vi "Get Indicators.vi"(6 "Indicator Names":string[](array[string]), 7 "Project Path":string, 8 "error in (no error)":errorcluster, 9 "VI Path":string, 10 "Target Name":string, 11 "tWorkerCommandRunner in":refnum<class "tWorkerCommandRunner.lvclass">) -> (0 "error out":errorcluster, 3 "tWorkerCommandRunner out":refnum<class "tWorkerCommandRunner.lvclass">)   [LabVIEW 2014, in "tWorkerCommandRunner.lvlib" / "tWorkerCommandRunner.lvclass"]
uses:
  tWorkerCommandRunner.lvclass
  BSON/tBSONDocument/tBSONDocument.lvclass
  <vilib>/ActorFramework/Actor/Actor.lvclass/Actor.ctl
  tWorkerTCPConnection/msgs/Return Run VI State Msg/Return Run VI State Msg.lvclass
  <vilib>/ActorFramework/Actor/Actor.lvclass
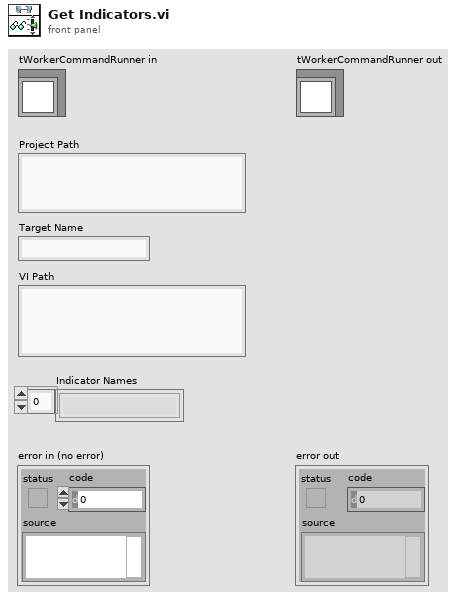
[diagram p1: front panel]
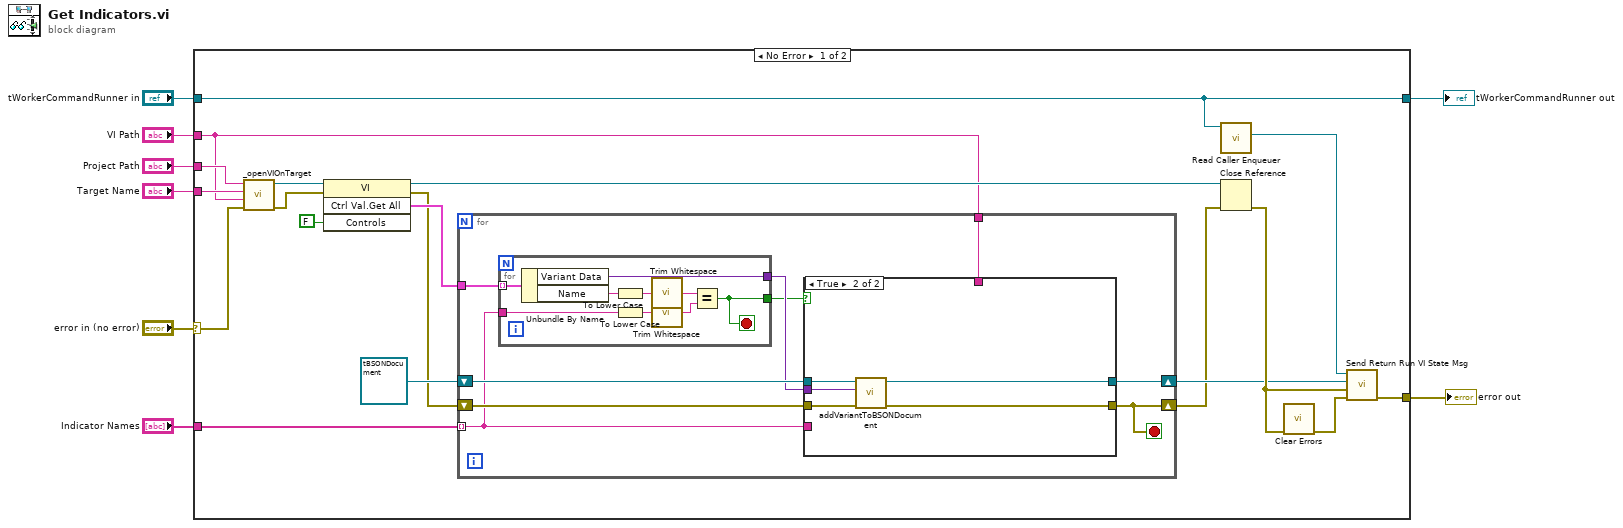
[diagram p0: block diagram]
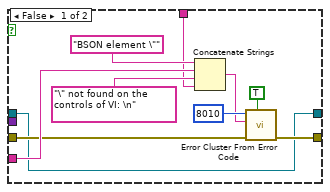
[diagram p2: hidden frame]
diagram:
  n1 = case shown="No Error" "error in (no error)" {
    selector: "error in (no error)" -> [w25 w62]
    tunnel: [w20 w62] -> w7
    tunnel: [w21 w61] -> w5
    tunnel: "tWorkerCommandRunner in" -> [w21 w61]
    tunnel: "VI Path" -> [w9 _]
    tunnel: "Project Path" -> [w27 _]
    tunnel: "Target Name" -> [w26 _]
    tunnel: "Indicator Names" -> [w13 _]
    frame No Error {
      n2 = call "_openVIOnTarget.vi"("error in (no error)"=w25, "VI Path"=w9, "Target Name"=w26, "Project Path"=w27) -> ("error out"=w14:errorcluster, "VI Reference"=w15:refnum<vi>)  [unwired: 6 in]
      n3 = invoke class="VI" method="Ctrl Val.Get All"(reference=w15, error in=w14, "Controls"=FALSE) -> (reference out=w11:refnum<vi>, error out=w16:errorcluster, "Get All Control Values Variant"=w18:cluster{"Name":string, "Variant Data":variant}[])  [unwired: 1 in, 1 out]
      n4 = for {
        tunnel: w18 -> [w36]
        shift-right: [w30] -> w12
        shift-left: refnum<class "tBSONDocument.lvclass"> refnum ("tBSONDocument in") -> [w35]
        shift-right: [w28] -> w10
        shift-left: w16 -> [w34]
        tunnel: w13 -> [w31] mode=indexing
        tunnel: w9 -> [w32]
        stop <- w28 stop-if-true
        n5 = for {
          tunnel: w36 -> [w60] mode=indexing
          tunnel: w31 -> [w58]
          tunnel: [w53] -> w33
          tunnel: [w52] -> w29
          stop <- w52 stop-if-true
          n6 = Unbundle By Name(w60) -> ("Variant Data"=w53:variant, "Name"=w59:string)
          n7 = To Lower Case(string=w59) -> (all lower case string=w57:string)
          n8 = To Lower Case(string=w58) -> (all lower case string=w56:string)
          n9 = call <vilib>:"Trim Whitespace.vi"("string"=w57) -> ("trimmed string"=w55:string)  [unwired: 1 in]
          n10 = call <vilib>:"Trim Whitespace.vi"("string"=w56) -> ("trimmed string"=w54:string)  [unwired: 1 in]
          n11 = Equal?(x=w55, y=w54) -> (x = y?=w52:bool)
        }
        n12 = case shown="True" w29 {
          tunnel: w31 -> [w42 _]
          tunnel: w32 -> [w40 _]
          tunnel: w35 -> [w37 w51]
          tunnel: w34 -> [w39 w50]
          tunnel: w33 -> [_ w49]
          tunnel: [w38 w48] -> w28
          tunnel: [w37 w47] -> w30
          frame False {
            n13 = Concatenate Strings("BSON element \"" ("string"), w42, "\" not found on the controls of VI: \n" ("string"), w40) -> (w43:string)
            n14 = call <vilib>:"Error Cluster From Error Code.vi"("show call chain? (False)"=TRUE, "error in (no error)"=w39, "error message (\"\")"=w43, "error code (0)"=8010) -> ("error out"=w38:errorcluster)  [unwired: 5 in]
          }
          frame True {
            n15 = call "addVariantToBSONDocument.vi"("error in (no error)"=w50, "Variant"=w49, "tBSONDocument in"=w51) -> ("error out"=w48:errorcluster, "tBSONDocument out"=w47:refnum<class "tBSONDocument.lvclass">)  [unwired: 7 in]
          }
        }
      }
      n16 = call <vilib>:"Read Caller Enqueuer.vi"("Actor"=w21) -> ("Caller Enqueuer"=w24:refnum<class "Message Enqueuer.lvclass">)  [unwired: 10 in]
      n17 = Close Reference(reference=w11, error in (no error)=w10) -> (error out=w23:errorcluster)
      n18 = call <vilib>:"Clear Errors.vi"("error in (no error)"=w23) -> ("error out"=w22:errorcluster)  [unwired: 5 in, 1 out]
      n19 = call "Send Return Run VI State Msg.vi"("error in (no error)"=w22, "Error From Run VI"=w23, "Indicators"=w12, "Message Enqueuer"=w24) -> ("error out"=w20:errorcluster)  [unwired: 6 in, 1 out]
    }
    frame Error {
    }
  }
  "error out" <- w7
  "tWorkerCommandRunner out" <- w5
